vi "Test Red-y Pressure Control CFG1.vi"(11 "Test Case In":refnum<class "Test Red-y Pressure Control CFG.lvclass">) -> (0 "error out":errorcluster, 3 "Test Case Out":refnum<class "Test Red-y Pressure Control CFG.lvclass">)   [LabVIEW 2023, in "Test Red-y Pressure Control CFG.lvclass"]
uses:
  Test Red-y Pressure Control CFG.lvclass
  C:/Program Files/National Instruments/LabVIEW 2023/vi.lib/Astemes/LUnit/Test Case.lvclass
  Measure and Stimulus Subsystems/Measure and Stimulus Subsystems.lvclass
  Virtual Instrs/Virt Red-y Read Write/Virt Red-y Read Write.lvclass
  Configurations/Pressure Control CFG/Red-y Pressure Control CFG.lvclass
  Configurations/Pressure Control CFG Simulated/Red-y Pressure Control CFG Simulated.lvclass
  <vilib>/Astemes/LUnit/Test Case.lvclass/Test Case.ctl
  <vilib>/Astemes/LUnit/Append Pass Result.vi
  <vilib>/Astemes/LUnit/Append Fail Result.vi
  <vilib>/Astemes/LUnit/Run In UI.vi
  <vilib>/Utility/error.llb/Clear Errors.vi
  Test Red-y Pressure Control CFG.lvclass/Test Red-y Pressure Control CFG.ctl
  <vilib>/Astemes/LUnit/Test Case.lvclass
  C:/Program Files/National Instruments/LabVIEW 2023/vi.lib/Astemes/LUnit/LUnit Runnable.lvclass
  D:/git/HAL/HAL GOOP4/Devices/Red-y/Tests/Test Red-y Pressure Control CFG/Test Red-y Pressure Control CFG.lvclass
panel:
  out "Pressure Scaling Max":variant
  out "Signal Type AI":variant
  out "Pressure":variant
  out "Output":variant
  out "Temperature":variant
  out "Flow":variant
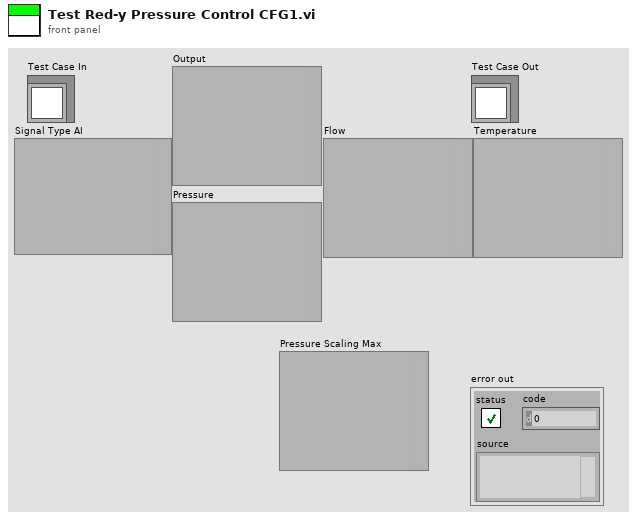
[diagram p1: front panel]
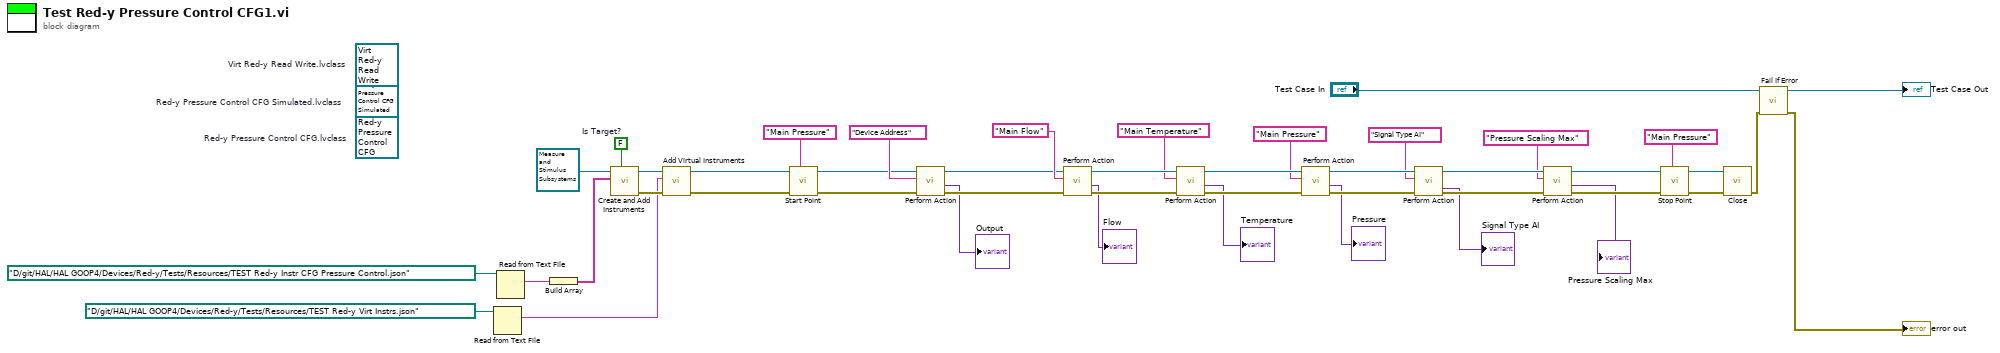
[diagram p0: block diagram]
diagram:
  (unwired) refnum<class "Red-y Pressure Control CFG Simulated.lvclass"> refnum  # Red-y Pressure Control CFG Simulated.lvclass
  (unwired) refnum<class "Red-y Pressure Control CFG.lvclass"> refnum  # Red-y Pressure Control CFG.lvclass
  (unwired) refnum<class "Virt Red-y Read Write.lvclass"> refnum  # Virt Red-y Read Write.lvclass
  w39 = FALSE  # Is Target?
  n1 = Read from Text File(file (use dialog)=path "D:/git/HAL/HAL GOOP4/Devices/Red-y/Tests/Resources/TEST Red-y Virt Instrs.json") -> (text=w1:string)  [unwired: 3 in, 3 out]
  n2 = Read from Text File(file (use dialog)=path "D:/git/HAL/HAL GOOP4/Devices/Red-y/Tests/Resources/TEST Red-y Instr CFG Pressure Control.json") -> (text=w3:string)  [unwired: 3 in, 3 out]
  n3 = Build Array(w3) -> (w38:string[])
  n4 = call "Create and Add Instruments.vi"("Is Target?"=w39, "Physical Intr CFGs"=w38, "MSS in"=refnum<class "Measure and Stimulus Subsystems.lvclass"> refnum ("HAL GOOP4.lvlib:Measure and Stimulus Subsystems.lvclass")) -> ("Error Out"=w41:errorcluster, "MSS out"=w40:refnum<class "Measure and Stimulus Subsystems.lvclass">)  [unwired: 6 in, 1 out]
  n5 = call "Add Virtual Instruments.vi"("error in"=w41, "<JSON CFG>"=w1, "MSS in"=w40) -> ("error out"=w37:errorcluster, "MSS out"=w21:refnum<class "Measure and Stimulus Subsystems.lvclass">)  [unwired: 6 in, 1 out]
  n6 = call "Start Point.vi"("Task-Point Ident"="Main Pressure", "error in"=w37, "MSS in"=w21) -> ("error out"=w22:errorcluster, "MSS out"=w20:refnum<class "Measure and Stimulus Subsystems.lvclass">)  [unwired: 7 in]
  n7 = call "Perform Action.vi"("error in"=w22, "Point Ident"="Device Address", "MSS in"=w20) -> ("error out"=w29:errorcluster, "Output"=→"Output":variant, "MSS out"=w28:refnum<class "Measure and Stimulus Subsystems.lvclass">)  [unwired: 5 in, 1 out]
  n8 = call "Perform Action.vi"("error in"=w29, "Point Ident"="Main Flow" ("Task-Point Idents"), "MSS in"=w28) -> ("error out"=w36:errorcluster, "Output"=→"Flow":variant, "MSS out"=w32:refnum<class "Measure and Stimulus Subsystems.lvclass">)  [unwired: 5 in, 1 out]
  n9 = call "Perform Action.vi"("error in"=w36, "Point Ident"="Main Temperature", "MSS in"=w32) -> ("error out"=w33:errorcluster, "Output"=→"Temperature":variant, "MSS out"=w24:refnum<class "Measure and Stimulus Subsystems.lvclass">)  [unwired: 5 in, 1 out]
  n10 = call "Perform Action.vi"("error in"=w33, "Point Ident"="Main Pressure", "MSS in"=w24) -> ("error out"=w25:errorcluster, "Output"=→"Pressure":variant, "MSS out"=w13:refnum<class "Measure and Stimulus Subsystems.lvclass">)  [unwired: 5 in, 1 out]
  n11 = call "Perform Action.vi"("error in"=w25, "Point Ident"="Signal Type AI", "MSS in"=w13) -> ("error out"=w14:errorcluster, "Output"=→"Signal Type AI":variant, "MSS out"=w9:refnum<class "Measure and Stimulus Subsystems.lvclass">)  [unwired: 5 in, 1 out]
  n12 = call "Perform Action.vi"("error in"=w14, "Point Ident"="Pressure Scaling Max", "MSS in"=w9) -> ("error out"=w10:errorcluster, "Output"=→"Pressure Scaling Max":variant, "MSS out"=w8:refnum<class "Measure and Stimulus Subsystems.lvclass">)  [unwired: 5 in, 1 out]
  n13 = call "Stop Point.vi"("Task-Point Idents"="Main Pressure", "error in"=w10, "MSS in"=w8) -> ("error out"=w18:errorcluster, "MSS out"=w17:refnum<class "Measure and Stimulus Subsystems.lvclass">)  [unwired: 7 in]
  n14 = call "Close.vi"("error in"=w18, "MSS in"=w17) -> ("error out"=w5:errorcluster)  [unwired: 8 in, 1 out]
  n15 = call <vilib>:"Fail If Error.vi"("error in (no error)"=w5, "LUnit Test Case In"="Test Case In") -> ("error out"=→"error out":errorcluster, "LUnit Test Case Out"=→"Test Case Out":refnum<class "Test Red-y Pressure Control CFG.lvclass">)  [unwired: 8 in]
